vi "Initialize.vi"(0 "Get PxlClk Slide":refnum<vi>, 5 "Get Expos Slide":refnum<vi>, 7 "Get FPS Slide":refnum<vi>, 9 "ROI Data Cluster":T1) -> (4 ".NET Refnum out":refnum<k24>, 6 "Camera SN":string, 8 "Bits/Pixel 2":i32, 15 "Error Out":errorcluster)   [LabVIEW 2021]
uses:
  C:/Program Files/Thorlabs/Scientific Imaging/ThorCam/uc480DotNet.dll
  Program Files/Thorlabs/Scientific Imaging/ThorCam/uc480DotNet.dll
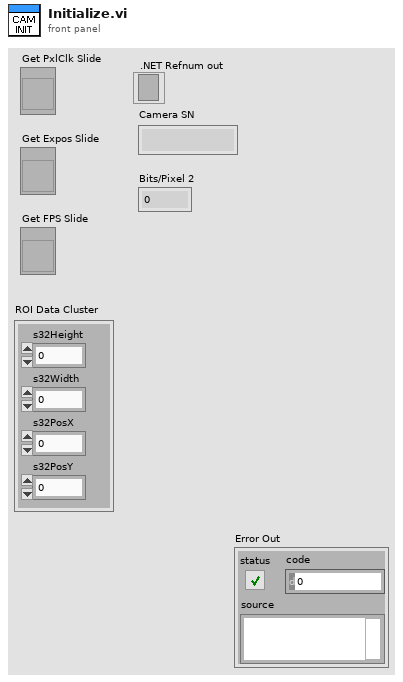
[diagram p1: front panel]
types:
  T1 = cluster{"s32PosX":i32, "s32PosY":i32, "s32Height":i32, "s32Width":i32}
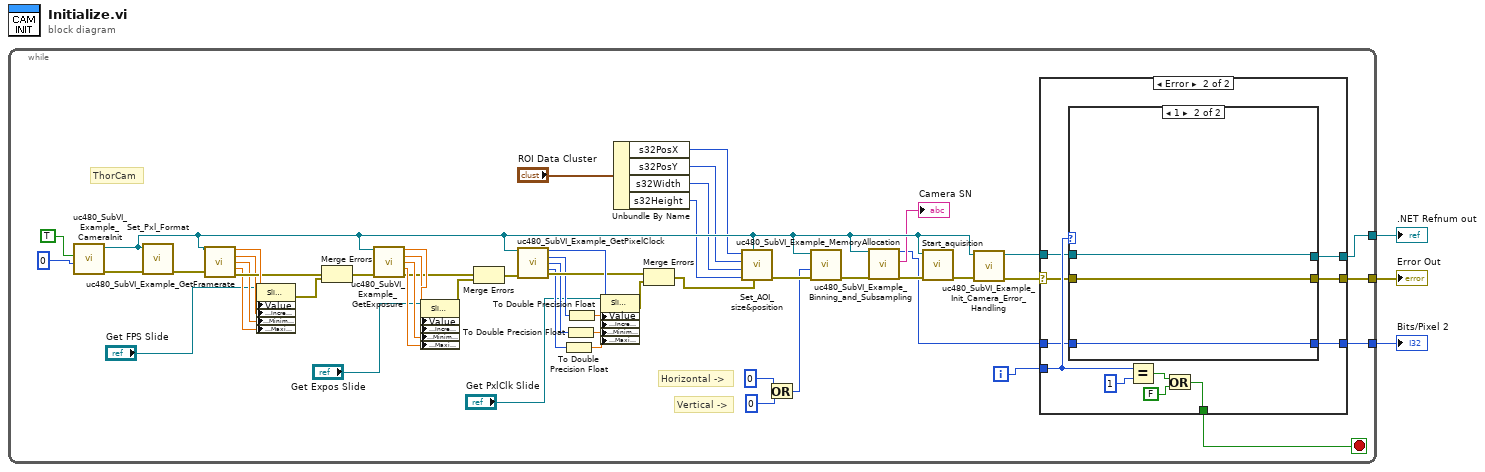
[diagram p0: block diagram]
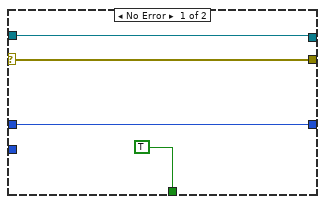
[diagram p2: hidden frame]
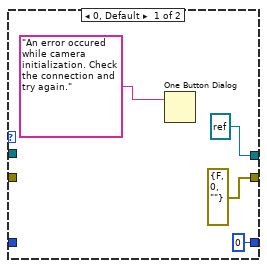
[diagram p3: hidden frame]
diagram:
  n1 = while {
    tunnel: [w7] -> w3
    tunnel: [w10] -> w2
    tunnel: [w8] -> w1
    i -> [w4]
    stop <- w5 stop-if-true
    # "ThorCam"
    # "Vertical ->"
    # "Horizontal ->"
    n2 = call "uc480_SubVI_Example_CameraInit.vi"("Camera ID"=0, "Init Camera Flag"=TRUE) -> ("Error Out"=w22:errorcluster, "uc480.Camera"=w56:refnum<k24>)  [unwired: 8 in]
    n3 = call "Set_Pxl_Format.vi"("error in (no error)"=w22, "uc480.Camera"=w56) -> ("error out"=w23:errorcluster)  [unwired: 9 in]
    n4 = call "uc480_SubVI_Example_GetFramerate.vi"("uc480.Camera"=w56, "Error In"=w23) -> ("Framerate"=w47:dbl, "Inc"=w32:dbl, "Min"=w33:dbl, "Max"=w34:dbl, "error out"=w35:errorcluster)  [unwired: 9 in]
    n5 = property on="Property Node" class="Slide (strict)"(reference="Get FPS Slide", "Value"=w47, "Scale.Increment"=w32, "Scale.Minimum"=w33, "Scale.Maximum"=w34) -> (error out=w36:errorcluster)  [unwired: 1 in, 1 out]
    n6 = Merge Errors(w35, w36) -> (w37:errorcluster)
    n7 = call "uc480_SubVI_Example_GetExposure.vi"("uc480.Camera"=w56, "Error In"=w37) -> ("Exposure"=w48:dbl, "Inc"=w28:dbl, "Min"=w29:dbl, "Max"=w30:dbl, "Error out"=w26:errorcluster)  [unwired: 9 in]
    n8 = property on="Property Node" class="Slide (strict)"(reference="Get Expos Slide", "Value"=w48, "Scale.Increment"=w28, "Scale.Minimum"=w29, "Scale.Maximum"=w30) -> (error out=w27:errorcluster)  [unwired: 1 in, 1 out]
    n9 = Merge Errors(w26, w27) -> (w31:errorcluster)
    n10 = call "uc480_SubVI_Example_GetPixelClock.vi"("uc480.Camera"=w56, "Error In"=w31) -> ("Pixel Clock"=w49:i32, "Inc"=w38:i32, "Min"=w40:i32, "Max"=w39:i32, "error out"=w44:errorcluster)  [unwired: 9 in]
    n11 = To Double Precision Float(number=w39) -> (double precision float=w43:dbl)
    n12 = To Double Precision Float(number=w40) -> (double precision float=w42:dbl)
    n13 = To Double Precision Float(number=w38) -> (double precision float=w41:dbl)
    n14 = property on="Property Node" class="Slide (strict)"(reference="Get PxlClk Slide", "Value"=w49, "Scale.Increment"=w41, "Scale.Minimum"=w42, "Scale.Maximum"=w43) -> (error out=w45:errorcluster)  [unwired: 1 in, 1 out]
    n15 = Unbundle By Name("ROI Data Cluster") -> ("s32PosX"=w15:i32, "s32PosY"=w12:i32, "s32Width"=w13:i32, "s32Height"=w14:i32)
    n16 = Merge Errors(w44, w45) -> (w52:errorcluster)
    n17 = call "Set_AOI_size&position.vi"("error in (no error)"=w52, "uc480.Camera"=w56, "s32Height"=w14, "s32Width"=w13, "s32PosY"=w12, "s32PosX"=w15) -> ("error out"=w53:errorcluster)  [unwired: 5 in]
    n18 = Or(x=0, y=0) -> (x .or. y?=w51:i32)
    n19 = call "uc480_SubVI_Example_Binning_and_Subsampling.vi"("Error In"=w53, "Subsampling Mode"=w51, "uc480.Camera"=w56) -> ("Error Out"=w50:errorcluster)  [unwired: 6 in, 2 out]
    n20 = call "uc480_SubVI_Example_MemoryAllocation.vi"("uc480.Camera"=w56, "Error In"=w50) -> ("Bits/Pixel 2"=w6:i32, "Serial Number"=→"Camera SN":string, "Error Out"=w24:errorcluster)  [unwired: 13 in, 2 out]
    n21 = call "Start_aquisition.vi"("error in (no error)"=w24, "uc480.Camera"=w56) -> ("error out"=w46:errorcluster)  [unwired: 8 in, 1 out]
    n22 = call "uc480_SubVI_Example_Init_Camera_Error_Handling.vi"("Error In"=w46, "uc480.Camera"=w56) -> ("Error Out"=w11:errorcluster, "uc480.Camera"=w9:refnum<k24>)  [unwired: 8 in]
    n23 = case shown="Error" w11 {
      selector: w11 -> [w60 w62]
      tunnel: [w60 w66] -> w10
      tunnel: w9 -> [w59 w63]
      tunnel: [w59 w65] -> w8
      tunnel: [w58 w67] -> w7
      tunnel: w6 -> [w58 w61]
      tunnel: [TRUE w69] -> w5
      tunnel: w4 -> [_ w64]
      frame No Error {
      }
      frame Error {
        n24 = case shown="1" w64 {
          tunnel: [0 ("Bits/Pixel 2") w76] -> w67
          tunnel: [errorcluster {"status"=FALSE, "code"=0, "source"=""} ("error IO") w77] -> w66
          tunnel: [refnum<k24> refnum ("uc480.Camera") w78] -> w65
          tunnel: w63 -> [_ w78]
          tunnel: w62 -> [_ w77]
          tunnel: w61 -> [_ w76]
          frame 0, Default {
            n25 = One Button Dialog(message="An error occured while camera initialization. Check the connection and try again.") -> ()  [unwired: 1 in, 1 out]
          }
          frame 1 {
          }
        }
        n26 = Equal?(x=w64, y=1) -> (x = y?=w70:bool)
        n27 = Or(x=w70, y=FALSE) -> (x .or. y?=w69:bool)
      }
    }
  }
  "Bits/Pixel 2" <- w3
  "Error Out" <- w2
  ".NET Refnum out" <- w1
